vi "ASI_CenterCalibration.vi"(8 "error in (no error)":errorcluster, 11 "VISA resource name":refnum<visa-resource-name>) -> (0 "error out":errorcluster, 3 "VISA resource name out":refnum<visa-resource-name>, 4 "y-range +-[mm]":dbl, 6 "x-range +-[mm]":dbl)   [LabVIEW 2011]
panel:
  out "+reached":bool
  out "-reached":bool
  out "set center string":string
  out "return move positive":string
  out "return move negative":string
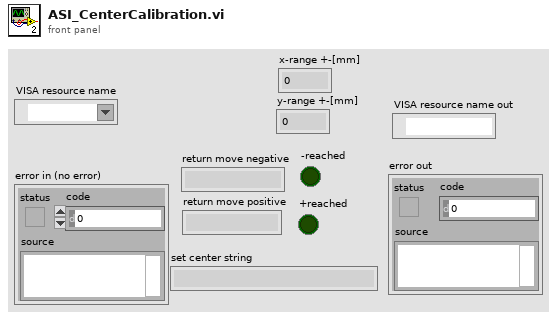
[diagram p1: front panel]
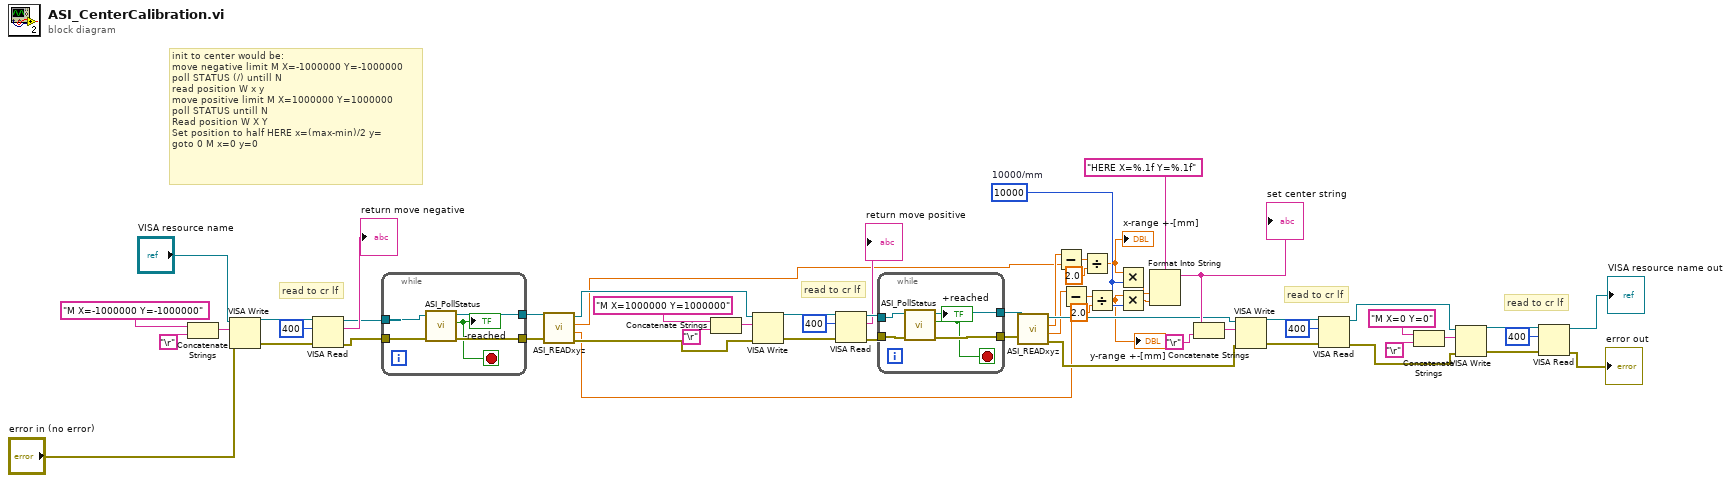
[diagram p0: block diagram]
diagram:
  w6 = 10000  # 10000/mm
  # "read to cr lf"
  # "read to cr lf"
  # "read to cr lf"
  # "init to center would be:\nmove negative limit M X=-1000000 Y=-1000000\npoll STATUS (/) untill N\nread position W x y\nmove positive limit M X=1000000 Y=1000000 \npoll STATUS untill N\nRead position W X Y\nSet position to half HERE x=(max-min)/2 y=\ngoto 0 M x=0 y=0"
  # "read to cr lf"
  n1 = Concatenate Strings("M X=-1000000 Y=-1000000" ("write buffer"), "\r") -> (w57:string)
  n2 = VISA Write(VISA resource name="VISA resource name", write buffer=w57, error in (no error)="error in (no error)") -> (VISA resource name out=w55:refnum<visa-resource-name>, error out=w52:errorcluster)  [unwired: 1 out]
  n3 = VISA Read(VISA resource name=w55, byte count=u32 400, error in (no error)=w52) -> (VISA resource name out=w49:refnum<visa-resource-name>, read buffer=→"return move negative":string, error out=w48:errorcluster)  [unwired: 1 out]
  n4 = while {
    tunnel: w49 -> [w63]
    tunnel: w48 -> [w62]
    tunnel: [w61] -> w46
    tunnel: [w60] -> w47
    stop <- w59 stop-if-true
    n5 = call "ASI_PollStatus.vi"("error in (no error)"=w62, "VISA resource name"=w63) -> ("error out"=w61:errorcluster, "Stopped"=w59:bool, "VISA resource name out"=w60:refnum<visa-resource-name>)  [unwired: 7 in]
    "-reached" <- w59
  }
  n6 = call "ASI_READxyz.vi"("error in (no error)"=w46, "VISA resource name"=w47) -> ("error out"=w38:errorcluster, "y [mm]"=w3:dbl, "x [mm]"=w12:dbl, "VISA resource name out"=w39:refnum<visa-resource-name>)  [unwired: 5 in, 1 out]
  n7 = Concatenate Strings("M X=1000000 Y=1000000" ("write buffer"), "\r") -> (w44:string)
  n8 = VISA Write(VISA resource name=w39, write buffer=w44, error in (no error)=w38) -> (VISA resource name out=w42:refnum<visa-resource-name>, error out=w40:errorcluster)  [unwired: 1 out]
  n9 = VISA Read(VISA resource name=w42, byte count=u32 400, error in (no error)=w40) -> (VISA resource name out=w37:refnum<visa-resource-name>, read buffer=→"return move positive":string, error out=w36:errorcluster)  [unwired: 1 out]
  n10 = while {
    tunnel: w37 -> [w68]
    tunnel: w36 -> [w67]
    tunnel: [w66] -> w33
    tunnel: [w65] -> w34
    stop <- w64 stop-if-true
    n11 = call "ASI_PollStatus.vi"("error in (no error)"=w67, "VISA resource name"=w68) -> ("error out"=w66:errorcluster, "Stopped"=w64:bool, "VISA resource name out"=w65:refnum<visa-resource-name>)  [unwired: 7 in]
    "+reached" <- w64
  }
  n12 = call "ASI_READxyz.vi"("error in (no error)"=w33, "VISA resource name"=w34) -> ("error out"=w27:errorcluster, "y [mm]"=w4:dbl, "x [mm]"=w13:dbl, "VISA resource name out"=w24:refnum<visa-resource-name>)  [unwired: 5 in, 1 out]
  n13 = Subtract(x=w13, y=w12) -> (x-y=w11:dbl)
  n14 = Subtract(x=w4, y=w3) -> (x-y=w8:dbl)
  n15 = Divide(x=w11, y=2.0) -> (x/y=w1:dbl)
  "x-range +-[mm]" <- w1
  n16 = Divide(x=w8, y=2.0) -> (x/y=w2:dbl)
  "y-range +-[mm]" <- w2
  n17 = Multiply(x=w1, y=w6) -> (x*y=w9:dbl)
  n18 = Multiply(x=w2, y=w6) -> (x*y=w5:dbl)
  n19 = Format Into String(format string="HERE X=%.1f Y=%.1f", w9, w5) -> (resulting string=w25:string)  [unwired: 2 in, 1 out]
  "set center string" <- w25
  n20 = Concatenate Strings(w25, "\r") -> (w31:string)
  n21 = VISA Write(VISA resource name=w24, write buffer=w31, error in (no error)=w27) -> (VISA resource name out=w30:refnum<visa-resource-name>, error out=w28:errorcluster)  [unwired: 1 out]
  n22 = VISA Read(VISA resource name=w30, byte count=u32 400, error in (no error)=w28) -> (VISA resource name out=w18:refnum<visa-resource-name>, error out=w17:errorcluster)  [unwired: 2 out]
  n23 = Concatenate Strings("M X=0 Y=0" ("write buffer"), "\r") -> (w23:string)
  n24 = VISA Write(VISA resource name=w18, write buffer=w23, error in (no error)=w17) -> (VISA resource name out=w21:refnum<visa-resource-name>, error out=w19:errorcluster)  [unwired: 1 out]
  n25 = VISA Read(VISA resource name=w21, byte count=u32 400, error in (no error)=w19) -> (VISA resource name out=→"VISA resource name out":refnum<visa-resource-name>, error out=→"error out":errorcluster)  [unwired: 2 out]
